vi "Start Nested.vi"(8 "error in (no error)":errorcluster caption="错误输入（无错误）", 11 "Actor in":refnum<class "RefNums and UICtrl.lvclass">) -> (0 "error out":errorcluster caption="错误输出", 3 "Actor out":refnum<class "RefNums and UICtrl.lvclass">)   [LabVIEW 2020, in "RefNums and UICtrl.lvclass"]
uses:
  RefNums and UICtrl.lvclass
  RefNums and UICtrl.lvclass/RefNums and UICtrl.ctl
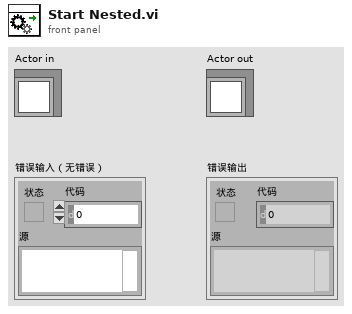
[diagram p1: front panel]
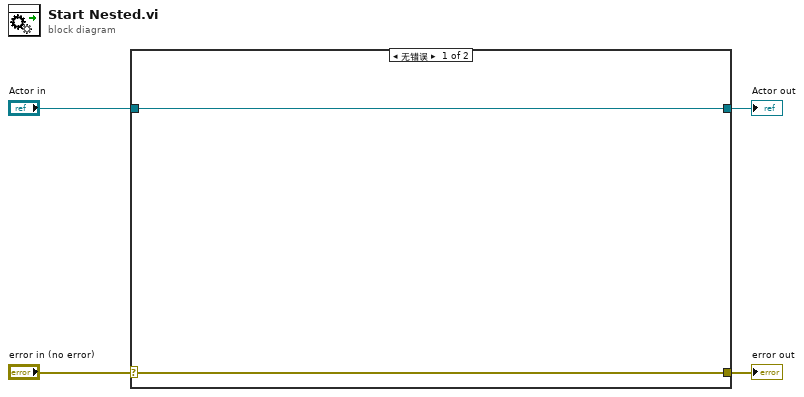
[diagram p0: block diagram]
diagram:
  n1 = case shown="无错误" "error in (no error)" {
    selector: "error in (no error)" -> [w5 w8]
    tunnel: [w5 w8] -> w3
    tunnel: [w6 w7] -> w1
    tunnel: "Actor in" -> [w6 w7]
    frame No Error {
    }
    frame Error {
    }
  }
  "error out" <- w3
  "Actor out" <- w1
